vi "Configure Channel.vi"(8 "error in (no error)":errorcluster, 10 "DAQmx Task In":refnum<k21>, 11 "DAQmxVoltageChannel in":refnum<class "VoltageInChannel.lvclass">) -> (0 "error out":errorcluster, 2 "DAQmx Task":refnum<k21>)   [LabVIEW 2020, in "VolatusDAQConfig.lvlib" / "VoltageInChannel.lvclass"]
uses:
  VoltageInChannel.lvclass
  VolatusConfig/Channel/Channel.lvclass
  C:/dev/lv20CE/relink/lv-volatus/VolatusDAQConfig/DAQmxChannel/DAQmxChannel.lvclass
  C:/dev/lv20CE/relink/lv-volatus/VolatusConfig/Channel/Channel.lvclass
  C:/dev/lv20CE/relink/lv-volatus/VolatusConfig/VolatusConfigElement/VolatusConfigElement.lvclass
  VolatusConfig/VolatusConfigElement/VolatusConfigElement.lvclass
  <vilib>/DAQmx/create/channels.llb/DAQmx Create Channel (AI-Voltage-Basic).vi
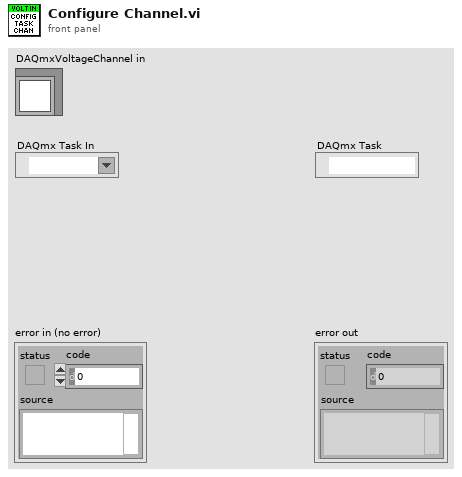
[diagram p1: front panel]
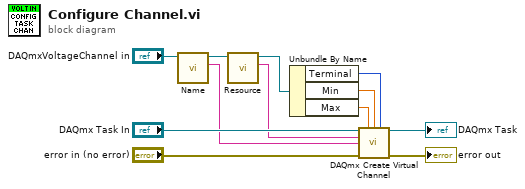
[diagram p0: block diagram]
diagram:
  n1 = call "Name.vi"("VolatusConfigElement in"="DAQmxVoltageChannel in") -> ("Name"=w1:string, "VolatusConfigElement out"=w2:refnum<class "VoltageInChannel.lvclass">)  [unwired: 8 in, 1 out]
  n2 = call "Resource.vi"("Channel in"=w2) -> ("Resource"=w3:string, "Channel out"=w4:refnum<class "VoltageInChannel.lvclass">)  [unwired: 8 in, 1 out]
  n3 = Unbundle By Name(w4) -> ("Terminal"=w7:i32, "Min"=w6:dbl, "Max"=w5:dbl)
  n4 = call-poly <vilib>:"DAQmx Create Virtual Channel.vi"("task in"="DAQmx Task In", "maximum value"=w5, "minimum value"=w6, "input terminal configuration"=w7, "physical channels"=w3, "name to assign"=w1, "error in"="error in (no error)") -> ("task out"=→"DAQmx Task":refnum<k21>, "error out"=→"error out":errorcluster)  [unwired: 7 in]
